vi "Analog Read.vi"   [LabVIEW 2011, in "LMH-LINX.lvlib"]
doc: "Read the value of the specified analog input channel(s)."
uses:
  LMH-LINX.lvlib
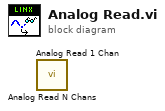
[diagram p0: block diagram]
diagram:
  n1 = call "Analog Read N Chans.vi"() -> ()  [unwired: 8 in, 4 out]
  n2 = call "Analog Read 1 Chan.vi"() -> ()  [unwired: 8 in, 4 out]
